vi "Is CSM Module - VIRef.vi"(8 "error in (no error)":errorcluster, 11 "VIRef":refnum<vi>) -> (0 "error out":errorcluster, 1 "CSMType":T1, 2 "Is CSM Module?":bool, 3 "CSM Basic Refs":T2)   [LabVIEW 2017, in "CSM-Helper Utility.lvlib"]
doc: "#### Is CSM Module - VIRef.vi\n\nDetermine if it is a CSM module through VIRef\n\n-- <b>Controls</b> --\n- <b>VIRef</b>: VI Reference\n\n-- <b>Indicators</b> --\n- <b>Is CSM Module?</b>: True If it is a CSM module\n- <b>CSM Basic Refs</b>: If This is a CSM module, It will return the basic references"
uses:
  CSM-Helper Utility.lvlib
  CSM Basic Refs.ctl
  CSM Module Type.ctl
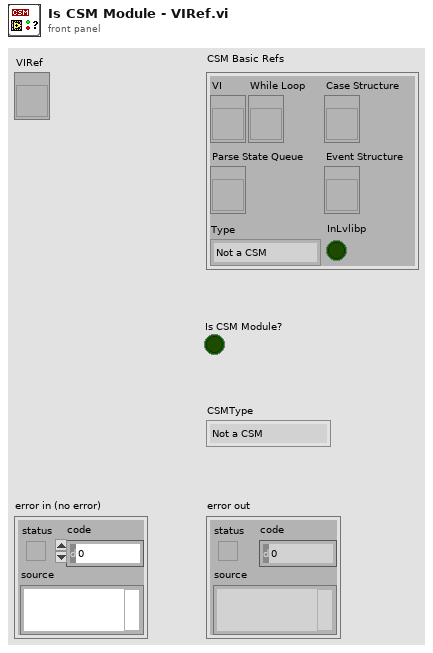
[diagram p1: front panel]
types:
  T1 = typedef "CSM-Helper Utility.lvlib/CSM Module Type.ctl" = enum16{"Not a CSM", "JKISM", "CSM"}
  T2 = typedef "CSM-Helper Utility.lvlib/CSM Basic Refs.ctl" = cluster{"VI":refnum<vi>, "While Loop":refnum<vi>, "Case Structure":refnum<vi>, "Parse State Queue":refnum<vi>, "Event Structure":refnum<vi>, "Type":T1, "InLvlibp":bool}
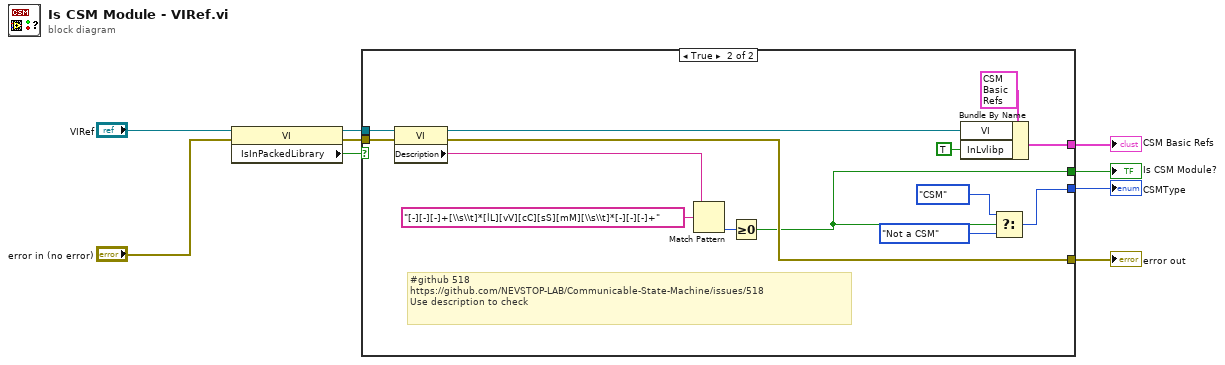
[diagram p0: block diagram]
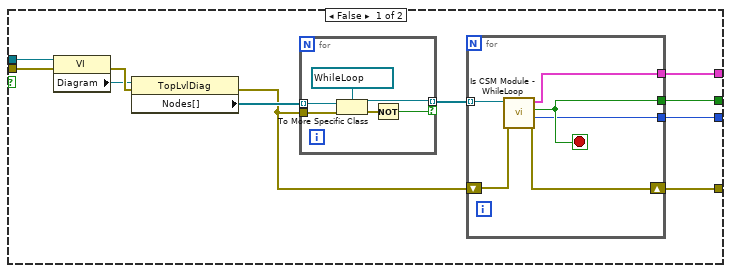
[diagram p2: hidden frame]
diagram:
  n1 = property class="VI"(reference="VIRef", error in="error in (no error)") -> (reference out=w4:refnum<vi>, error out=w3:errorcluster, "IsInPackedLibrary"=w1:bool)
  n2 = case shown="True" w1 {
    tunnel: [w16 w34] -> w8
    tunnel: [w14 w45] -> w7
    tunnel: [w13 w38] -> w6
    tunnel: [w12 w35] -> w5
    tunnel: w4 -> [w11 w44]
    tunnel: w3 -> [w10 w43]
    frame False {
      n3 = property on="Property Node" class="VI"(reference=w11, error in=w10) -> (error out=w20:errorcluster, "Diagram"=w18:refnum<vi>)  [unwired: 1 out]
      n4 = property on="Property Node" class="TopLvlDiag"(reference=w18, error in=w20) -> (error out=w15:errorcluster, "Nodes[]"=w19:refnum<vi>[])  [unwired: 1 out]
      n5 = for {
        tunnel: w19 -> [w31] mode=indexing
        tunnel: [w29] -> w17 mode=indexing if=w27
        tunnel: w15 -> [w30]
        n6 = To More Specific Class(target class=refnum<vi> refnum ("WLoop Refnum"), reference=w31, error in=w30) -> (specific class reference=w29:refnum<vi>, error out=w28:errorcluster)
        n7 = Not(x=w28) -> (.not. x?=w27:bool)
      }
      n8 = for {
        tunnel: w17 -> [w23] mode=indexing
        tunnel: [w24] -> w16
        tunnel: [w22] -> w14
        tunnel: [w21] -> w12
        shift-right: [w26] -> w13
        shift-left: w15 -> [w25]
        stop <- w24 stop-if-true
        n9 = call "Is CSM Module - WhileLoop.vi"("error in (no error)"=w25, "WhileLoop in"=w23) -> ("error out"=w26:errorcluster, "CSMType"=w21:T1, "Is CSM Module?"=w24:bool, "CSM Basic Refs"=w22:T2)  [unwired: 6 in]
      }
    }
    frame True {
      # "#github 518  \nhttps://github.com/NEVSTOP-LAB/Communicable-State-Machine/issues/518\nUse description to check"
      n10 = property class="VI"(reference=w44, error in=w43) -> (reference out=w42:refnum<vi>, error out=w38:errorcluster, "Description"=w41:string)
      n11 = Match Pattern(string=w41, regular expression="[-][-][-]+[\\s\\t]*[lL][vV][cC][sS][mM][\\s\\t]*[-][-][-]+") -> (offset past match=w39:i32)  [unwired: 1 in, 3 out]
      n12 = Greater Or Equal To 0?(x=w39) -> (x >= 0?=w34:bool)
      n13 = Bundle By Name(cluster=T2 {"VI"=refnum, "While Loop"=refnum, "Case Structure"=refnum, "Parse State Queue"=refnum, "Event Structure"=refnum, "Type"=enum."Not a CSM", "InLvlibp"=FALSE} ("CSM Basic Refs"), "VI"=w42, "InLvlibp"=TRUE) -> (w45:T2)
      n14 = Select(t=CSM_Module_Type."CSM" ("CSMType"), s=w34, f=CSM_Module_Type."Not a CSM" ("CSMType")) -> (s? t:f=w35:T1)
    }
  }
  "error out" <- w6
  "Is CSM Module?" <- w8
  "CSM Basic Refs" <- w7
  "CSMType" <- w5
